vi "SQL.TestData.vi"(3 "最大查询天数":u32, 5 "单项查询索引":i32, 6 "error in (no error)":errorcluster, 7 "Folder Path":path caption="文件夹路径", 8 "Result":string, 9 "Serial_number":string, 10 "Time":string, 11 "Date":string) -> (0 "SQL Results":string[][](table)=[["1.Audio RX", "91.081303", "2.Audio TX", "0.095270", "20121122", "13:32:50", "1170000000689", "PASS"], ["1.Audio RX", "91.143105", "2.Audio TX", "0.095494", "20121122", "13:39:33", "1170000000689", "PASS"], ["1.Audio RX", "91.991153", "2.Audio TX", "0.100831", "20121122", "13:54:04", "1111111111111", "PASS"], ["1.Audio RX", "91.857442", "2.Audio TX", "0.105589", "20121122", "13:56:23", "1172000000041", "PASS"], ["1.Audio RX", "92.085102", "2.Audio TX", "0.101190", "20121122", "13:57:37", "1172000000027", "PASS"], ["1.Audio RX", "91.878361", "2.Audio TX", "0.100191", "20121122", "13:59:11", "1172000000362", "PASS"], ["1.Audio RX", "92.029742", "2.Audio TX", "0.098333", "20121122", "14:02:06", "1172000000287", "PASS"], ["1.Audio RX", "91.480339", "2.Audio TX", "0.101565", "20121122", "14:04:55", "1170000000436", "PASS"], ["1.Audio RX", "91.969090", "2.Audio TX", "0.101169", "20121122", "14:06:27", "1172000000171", "PASS"], ["1.Audio RX", "92.221462", "2.Audio TX", "0.099581", "20121122", "14:09:34", "1172000000034", "PASS"], ["1.Audio RX", "91.987652", "2.Audio TX", "0.098084", "20121122", "14:11:36", "1172000000317", "PASS"], ["1.Audio RX", "92.074553", "2.Audio TX", "0.099366", "20121122", "14:13:21", "1172000000263", "PASS"], ["1.Audio RX", "92.132843", "2.Audio TX", "0.098619", "20121122", "14:14:51", "1172000000492", "PASS"], ["1.Audio RX", "92.082562", "2.Audio TX", "0.099291", "20121122", "14:16:15", "1172000000010", "PASS"], ["1.Audio RX", "91.950055", "2.Audio TX", "0.100073", "20121122", "14:17:31", "1172000000041", "PASS"], ["1.Audio RX", "92.103586", "2.Audio TX", "0.100658", "20121122", "14:28:07", "0000000000000", "PASS"], ["1.Audio RX", "92.130135", "2.Audio TX", "0.099393", "20121122", "14:31:21", "1172000000331", "PASS"], ["1.Audio RX", "92.260601", "2.Audio TX", "0.099085", "20121122", "14:33:09", "1172000000416", "PASS"], ["1.Audio RX", "91.917260", "2.Audio TX", "0.099118", "20121122", "14:34:45", "1172000000294", "PASS"], ["1.Audio RX", "91.905751", "2.Audio TX", "0.097974", "20121122", "14:36:10", "1172000000423", "PASS"], ["1.Audio RX", "92.133605", "2.Audio TX", "0.097918", "20121122", "14:37:41", "1172000000119", "PASS"], ["1.Audio RX", "92.096734", "2.Audio TX", "0.102493", "20121122", "14:40:09", "1172000000508", "PASS"], ["1.Audio RX", "92.042766", "2.Audio TX", "0.097988", "20121122", "14:41:47", "1172000000157", "PASS"], ["1.Audio RX", "92.072530", "2.Audio TX", "0.098405", "20121122", "14:42:41", "1172000000157", "PASS"], ["1.Audio RX", "91.988608", "2.Audio TX", "0.100953", "20121122", "14:45:30", "1172000000164", "PASS"], ["1.Audio RX", "92.115288", "2.Audio TX", "0.099866", "20121122", "14:46:43", "1172000000379", "PASS"], ["1.Audio RX", "91.931552", "2.Audio TX", "0.098401", "20121122", "14:48:07", "1172000000201", "PASS"], ["1.Audio RX", "92.141466", "2.Audio TX", "0.102419", "20121122", "14:49:20", "1172000000324", "PASS"], ["1.Audio RX", "91.932576", "2.Audio TX", "0.099878", "20121122", "14:51:57", "1172000000355", "PASS"], ["1.Audio RX", "92.147045", "2.Audio TX", "0.096185", "20121122", "14:54:23", "1172000000133", "PASS"], ["1.Audio RX", "92.010262", "2.Audio TX", "0.097653", "20121122", "14:55:55", "1172000000270", "PASS"], ["1.Audio RX", "92.200920", "2.Audio TX", "0.099317", "20121122", "14:57:32", "1172000000065", "PASS"], ["1.Audio RX", "92.066286", "2.Audio RX", "91.980270", "20121122", "15:11:29", "", "PASS"], ["1.Audio RX", "92.152783", "2.Audio RX", "92.048697", "20121122", "15:14:00", "", "PASS"], ["1.Audio RX", "92.058673", "2.Audio TX", "0.099819", "20121122", "15:54:48", "1170000000689", "PASS"], ["1.Audio RX", "91.953046", "2.Audio TX", "0.099171", "20121122", "15:58:55", "1170000000436", "PASS"]], 1 "单项数据结果":string[](array[string]), 4 "error out":errorcluster)   [LabVIEW 2012, in "Lib_UEL.ATE.lvlib" / "Lib_SQL.lvlib"]
uses:
  Lib_SQL.lvlib
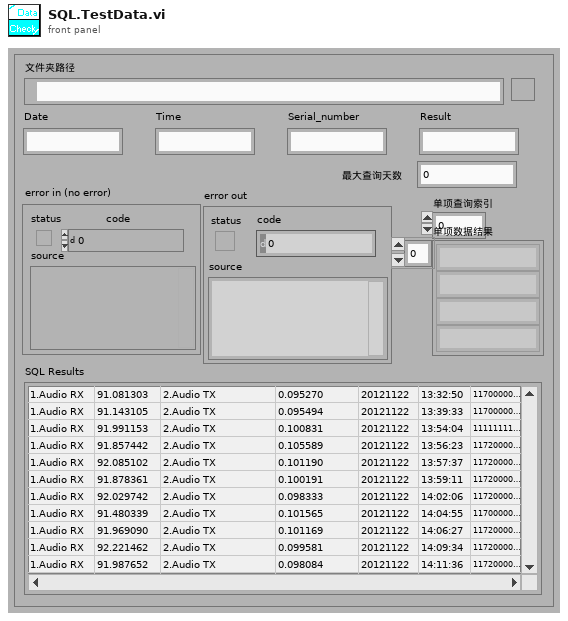
[diagram p1: front panel]
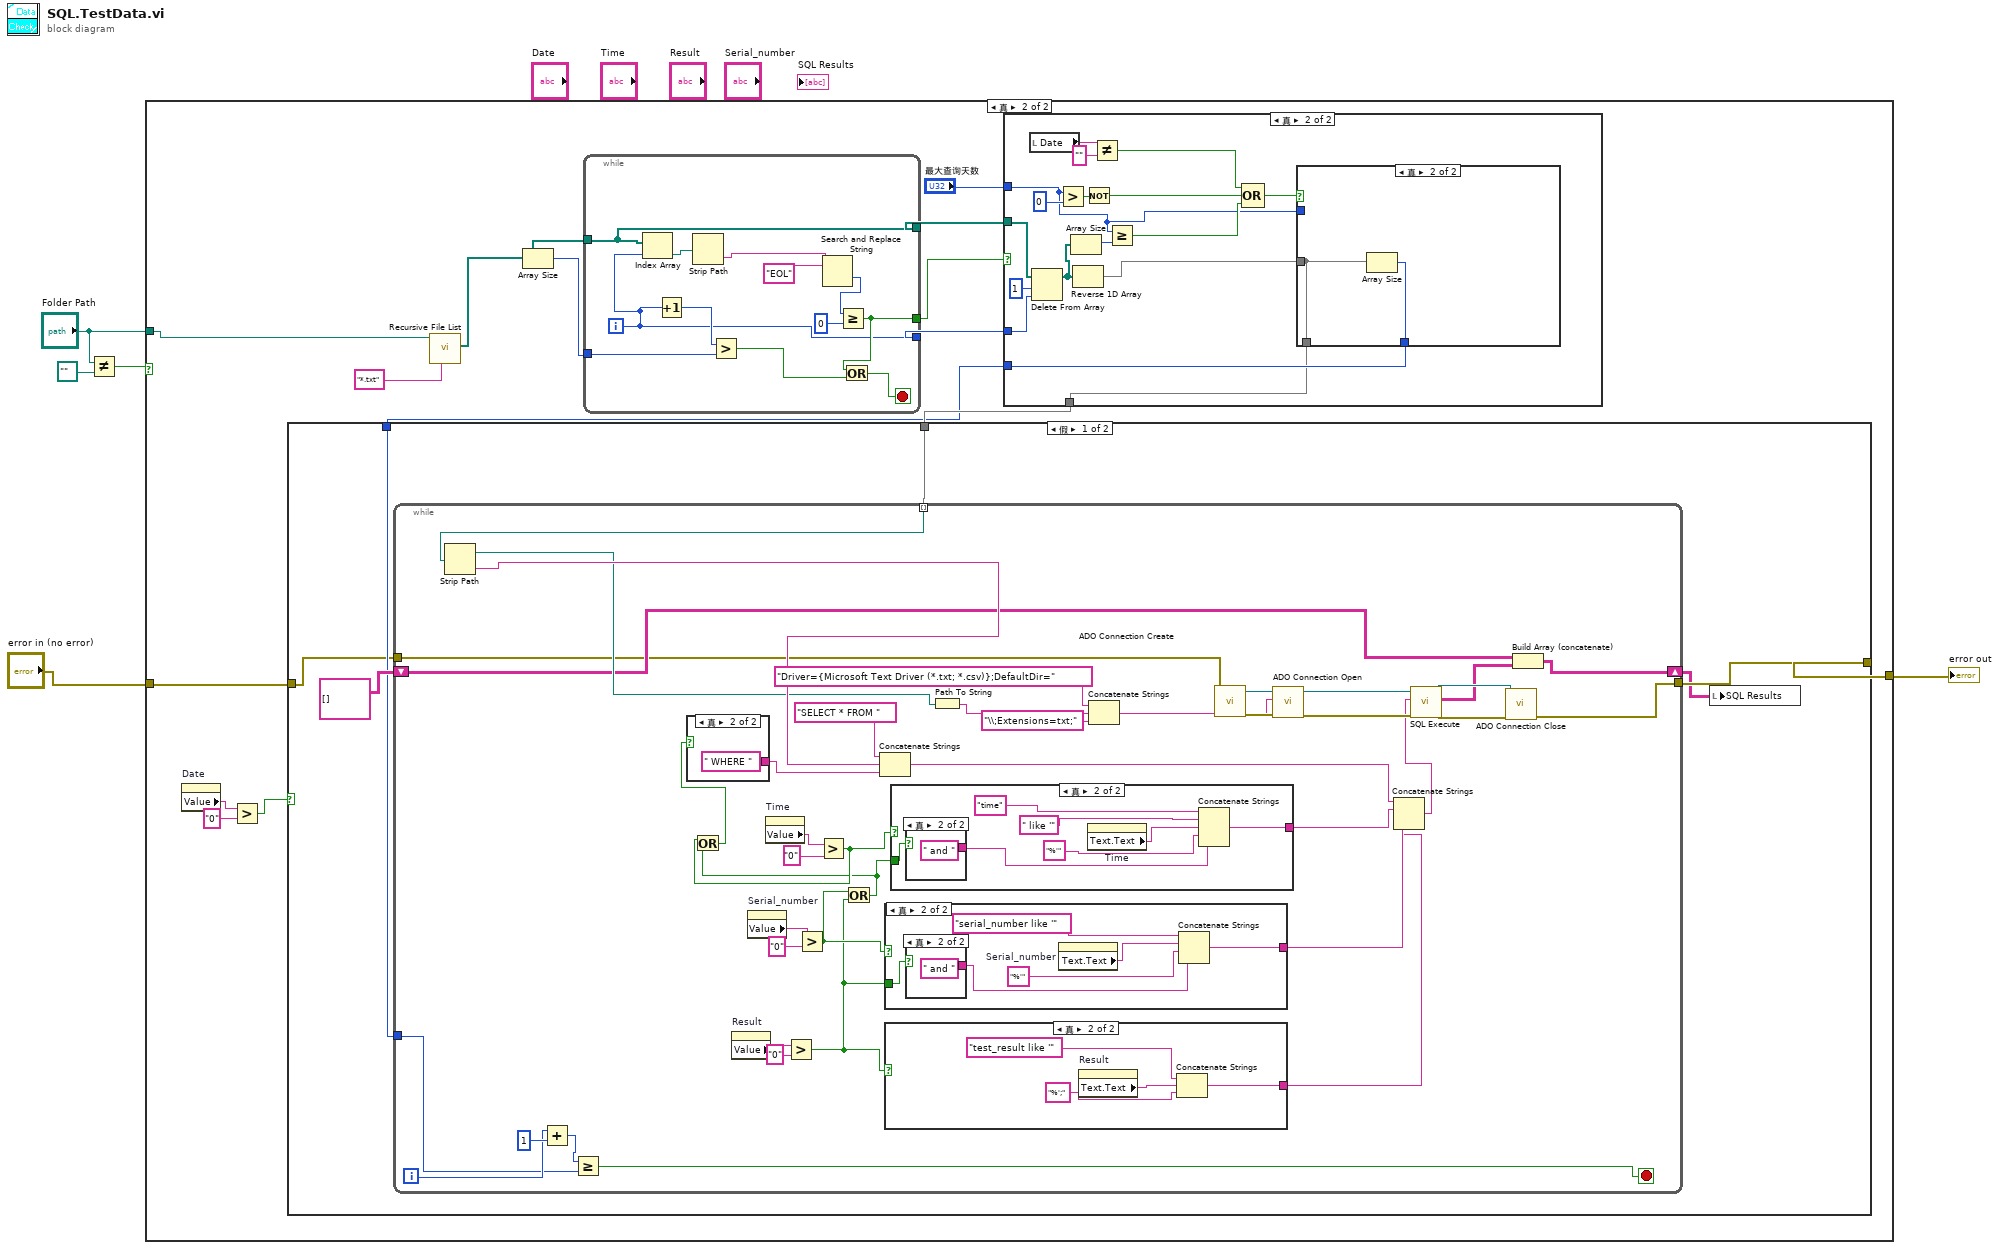
[diagram p0: block diagram]
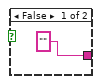
[diagram p3: hidden frame]
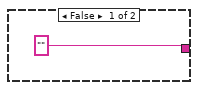
[diagram p4: hidden frame]
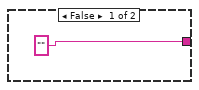
[diagram p5: hidden frame]
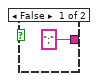
[diagram p6: hidden frame]
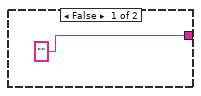
[diagram p7: hidden frame]
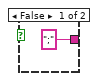
[diagram p8: hidden frame]
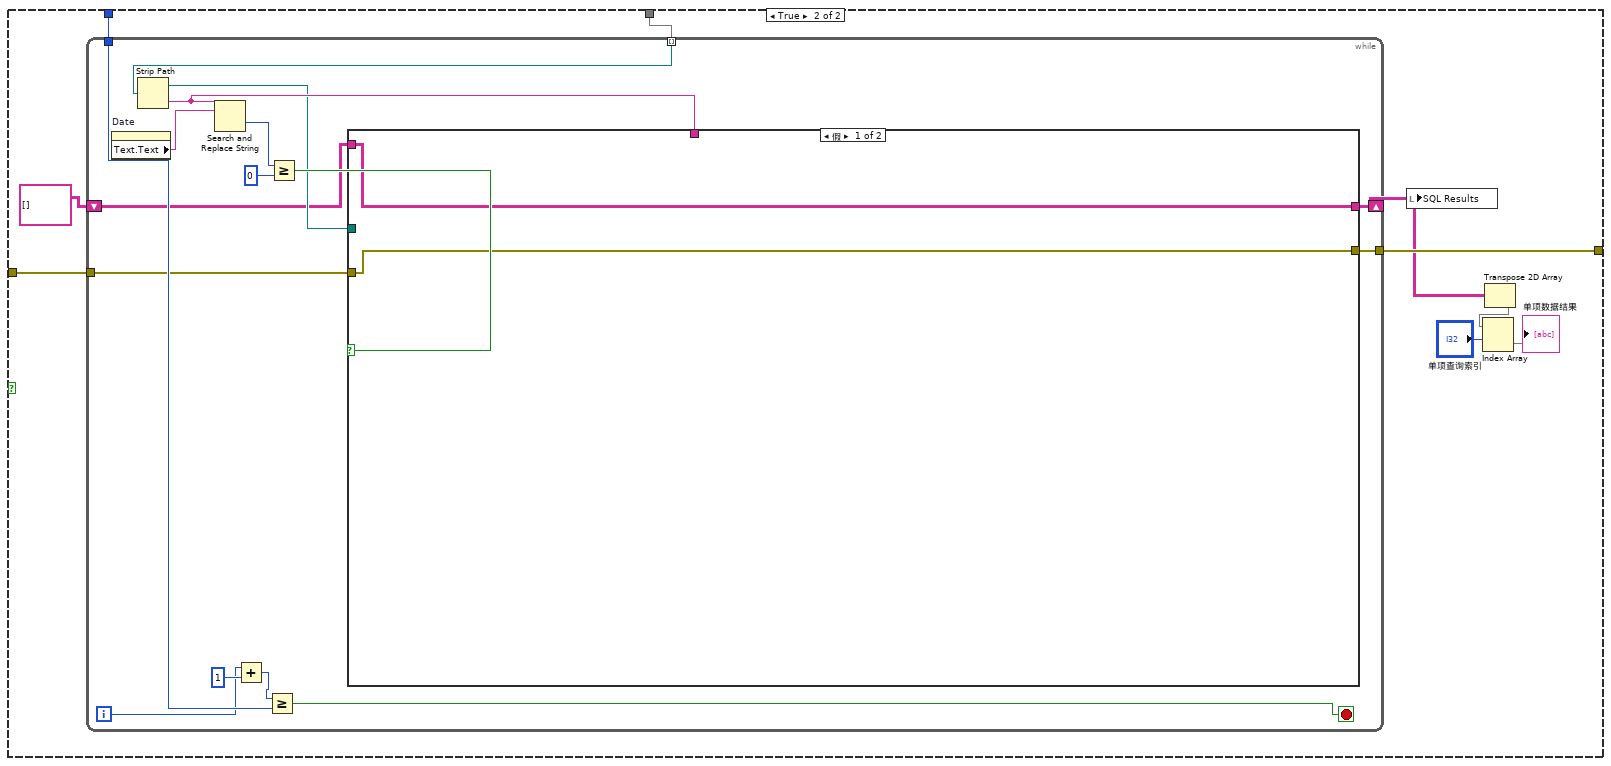
[diagram p9: hidden frame]
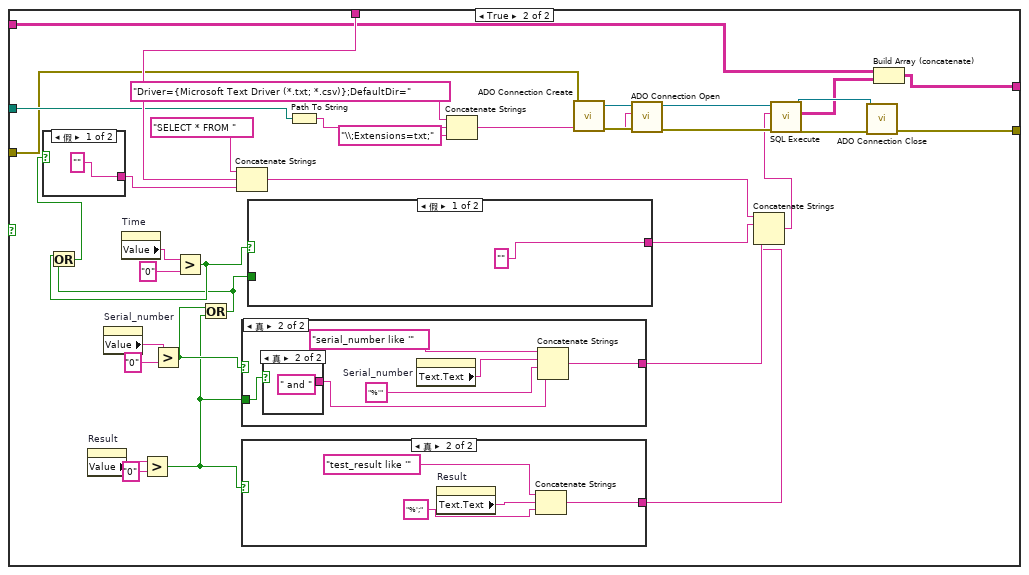
[diagram p10: hidden frame]
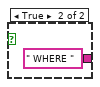
[diagram p11: hidden frame]
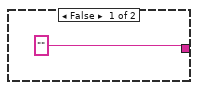
[diagram p12: hidden frame]
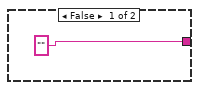
[diagram p13: hidden frame]
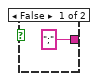
[diagram p14: hidden frame]
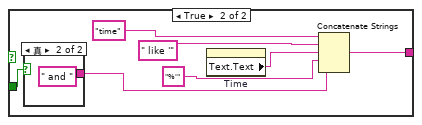
[diagram p15: hidden frame]
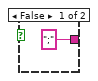
[diagram p16: hidden frame]
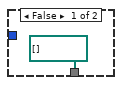
[diagram p17: hidden frame]
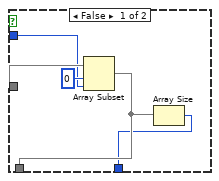
[diagram p18: hidden frame]
diagram:
  n1 = Not Equal?(x="Folder Path", y=path "") -> (x != y?=w1:bool)
  n2 = case shown="真" w1 {
    tunnel: "Folder Path" -> [_ w21]
    tunnel: [w6 w11] -> w5
    tunnel: "error in (no error)" -> [w6 w9]
    frame False {
    }
    frame True {
      n3 = property on="Date" class="Str"() -> ("Value"=w15:string)  [unwired: 2 in, 2 out]
      n4 = Greater?(x=w15, y="0") -> (0:w13:bool)
      n5 = call <vilib>:"Recursive File List.vi"("pattern"="*.txt", "Folder Path"=w21) -> ("All Files in Dir"=w8:path[])  [unwired: 5 in, 4 out]
      n6 = Array Size(array=w8) -> (size(s)=w7:i32)
      n7 = while {
        tunnel: w8 -> [w211]
        tunnel: [w211] -> w19
        tunnel: w7 -> [w210]
        tunnel: [w209] -> w18
        tunnel: [w208] -> w17
        i -> [w208]
        stop <- w212 stop-if-true
        n8 = Index Array(array=w211, index=w208) -> (element=w214:path)
        n9 = Increment(x=w208) -> (x+1=w218:i32)
        n10 = Strip Path(path=w214) -> (name=w213:string)  [unwired: 1 out]
        n11 = Greater?(x=w218, y=w210) -> (0:w215:bool)
        n12 = Search and Replace String(input string=w213, search string="EOL" ("搜索字符串")) -> (offset past replacement=w217:i32)  [unwired: 6 in, 3 out]
        n13 = Greater Or Equal?(x=w217, y=0) -> (x >= y?=w209:bool)
        n14 = Or(x=w209, y=w215) -> (x .or. y?=w212:bool)
      }
      n15 = case shown="真" w18 {
        tunnel: w19 -> [_ w199]
        tunnel: w17 -> [_ w198]
        tunnel: [path[] [] ("All Files in Dir") w195] -> w16
        tunnel: [_ w197] -> w12
        tunnel: "最大查询天数" -> [_ w187]
        frame False {
        }
        frame True {
          n16 = local read "Date"() -> (w186:string)
          n17 = Delete From Array(array=w199, length=1 ("长度"), index=w198) -> (array with subset deleted=w193:path[])  [unwired: 1 out]
          n18 = Greater?(x=w187, y=u32 0) -> (0:w189:bool)
          n19 = Array Size(array=w193) -> (size(s)=w192:i32)
          n20 = Reverse 1D Array(array=w193) -> (reversed array=w194:path[])
          n21 = Not(x=w189) -> (.not. x?=w188:bool)
          n22 = Not Equal?(x=w186, y="") -> (x != y?=w184:bool)
          n23 = Greater Or Equal?(x=w187, y=w192) -> (x >= y?=w190:bool)
          n24 = Compound Arithmetic op=OR(w184, w188, w190) -> (w191:bool)
          n25 = case shown="真" w191 {
            tunnel: w194 -> [w205 w206]
            tunnel: [w201 w207] -> w197
            tunnel: [w202 w206] -> w195
            tunnel: w187 -> [w203 _]
            frame False {
              n26 = Array Subset(array=w205, index=0 ("索引"), length=w203) -> (w202:path[])
              n27 = Array Size(array=w202) -> (size(s)=w201:i32)
            }
            frame True {
              n28 = Array Size(array=w206) -> (size(s)=w207:i32)
            }
          }
        }
      }
      n29 = case shown="假" w13 {
        tunnel: w16 -> [w26 w103]
        tunnel: w12 -> [w25 w102]
        tunnel: [w24 w100] -> w11
        tunnel: w9 -> [w23 w99]
        frame False {
          n30 = while {
            tunnel: w26 -> [w67] mode=indexing
            shift-right: [w60] -> w22
            shift-left: string[][] [] ("Data") -> [w61]
            tunnel: w25 -> [w59]
            tunnel: [w29] -> w24
            tunnel: w23 -> [w28]
            i -> [w63]
            stop <- w64 stop-if-true
            n31 = Strip Path(path=w67) -> (stripped path=w62:path, name=w68:string)
            n32 = Add(x=w63, y=1) -> (x+y=w66:i32)
            n33 = Greater Or Equal?(x=w66, y=w59) -> (x >= y?=w64:bool)
            n34 = property on="Result" class="Str"() -> ("Value"=w43:string)  [unwired: 2 in, 2 out]
            n35 = property on="Serial_number" class="Str"() -> ("Value"=w45:string)  [unwired: 2 in, 2 out]
            n36 = property on="Time" class="Str"() -> ("Value"=w47:string)  [unwired: 2 in, 2 out]
            n37 = Greater?(x=w43, y="0") -> (0:w34:bool)
            n38 = Greater?(x=w45, y="0") -> (0:w35:bool)
            n39 = Greater?(x=w47, y="0") -> (0:w32:bool)
            n40 = Or(x=w35, y=w34) -> (x .or. y?=w31:bool)
            n41 = Or(x=w32, y=w31) -> (x .or. y?=w33:bool)
            n42 = case shown="真" w33 {
              tunnel: ["" " WHERE "] -> w41
              frame False {
              }
              frame True {
              }
            }
            n43 = Concatenate Strings("SELECT * FROM ", w68, w41) -> (w40:string)
            n44 = case shown="真" w35 {
              tunnel: ["" w78] -> w38
              tunnel: w34 -> [_ w77]
              frame False {
              }
              frame True {
                n45 = case shown="真" w77 {
                  tunnel: [";" " and "] -> w79
                  frame False {
                  }
                  frame True {
                  }
                }
                n46 = property on="Serial_number" class="Str"() -> ("Text.Text"=w81:string)  [unwired: 2 in, 2 out]
                n47 = Concatenate Strings("serial_number like '", w81, "%'", w79) -> (w78:string)
              }
            }
            n48 = case shown="真" w34 {
              tunnel: ["" w72] -> w37
              frame False {
              }
              frame True {
                n49 = property on="Result" class="Str"() -> ("Text.Text"=w74:string)  [unwired: 2 in, 2 out]
                n50 = Concatenate Strings("test_result like '", w74, "%';") -> (w72:string)
              }
            }
            n51 = case shown="真" w32 {
              tunnel: ["" w87] -> w39
              tunnel: w31 -> [_ w86]
              frame False {
              }
              frame True {
                n52 = case shown="真" w86 {
                  tunnel: [";" " and "] -> w88
                  frame False {
                  }
                  frame True {
                  }
                }
                n53 = property on="Time" class="Str"() -> ("Text.Text"=w90:string)  [unwired: 2 in, 2 out]
                n54 = Concatenate Strings("time", " like '", w90, "%'", w88) -> (w87:string)
              }
            }
            n55 = Path To String(path=w62) -> (string=w50:string)
            n56 = Concatenate Strings("Driver={Microsoft Text Driver (*.txt; *.csv)};DefaultDir=", w50, "\\;Extensions=txt;" ("字符串")) -> (w48:string)
            n57 = call <userlib>:"ADO Connection Create.vi"("error in (no error)"=w28) -> ("error out"=w56:errorcluster, "ADODB._Connection Out"=w57:refnum<k7>)  [unwired: 9 in]
            n58 = call <userlib>:"ADO Connection Open.vi"("error in (no error)"=w56, "ConnectionString"=w48, "ADODB._Connection In"=w57) -> ("error out"=w54:errorcluster, "ADODB._Connection Out"=w55:refnum<k7>)  [unwired: 7 in]
            n59 = Concatenate Strings(w40, w39, w38, w37) -> (w36:string)
            n60 = call <userlib>:"SQL Execute.vi"("error in (no error)"=w54, "Command Text"=w36, "ADODB._Connection In"=w55) -> ("error out"=w53:errorcluster, "Data"=w30:string[][], "ADODB._Connection Out"=w52:refnum<k7>)  [unwired: 5 in, 1 out]
            n61 = call <userlib>:"ADO Connection Close.vi"("error in (no error)"=w53, "ADODB._Connection In"=w52) -> ("error out"=w29:errorcluster)  [unwired: 8 in, 1 out]
            n62 = Build Array (concatenate)(w61, w30) -> (w60:string[][])
          }
          n63 = local write "SQL Results"(w22) -> ()
        }
        frame True {
          n64 = while {
            tunnel: w103 -> [w116] mode=indexing
            tunnel: w102 -> [w115]
            shift-right: [w106] -> w95
            shift-left: string[][] [] ("Data") -> [w107]
            tunnel: [w105] -> w100
            tunnel: w99 -> [w104]
            i -> [w109]
            stop <- w110 stop-if-true
            n65 = property on="Date" class="Str"() -> ("Text.Text"=w114:string)  [unwired: 2 in, 2 out]
            n66 = Strip Path(path=w116) -> (stripped path=w108:path, name=w117:string)
            n67 = Search and Replace String(input string=w117, search string=w114) -> (offset past replacement=w119:i32)  [unwired: 6 in, 3 out]
            n68 = Add(x=w109, y=1) -> (x+y=w112:i32)
            n69 = Greater Or Equal?(x=w112, y=w115) -> (x >= y?=w110:bool)
            n70 = Greater Or Equal?(x=w119, y=0) -> (x >= y?=w118:bool)
            n71 = case shown="假" w118 {
              tunnel: w117 -> [_ w155]
              tunnel: w108 -> [_ w127]
              tunnel: [w121 w124] -> w106
              tunnel: w107 -> [w121 w126]
              tunnel: [w120 w123] -> w105
              tunnel: w104 -> [w120 w122]
              frame False {
              }
              frame True {
                n72 = property on="Result" class="Str"() -> ("Value"=w140:string)  [unwired: 2 in, 2 out]
                n73 = property on="Serial_number" class="Str"() -> ("Value"=w142:string)  [unwired: 2 in, 2 out]
                n74 = property on="Time" class="Str"() -> ("Value"=w144:string)  [unwired: 2 in, 2 out]
                n75 = Greater?(x=w140, y="0") -> (0:w131:bool)
                n76 = Greater?(x=w142, y="0") -> (0:w132:bool)
                n77 = Greater?(x=w144, y="0") -> (0:w129:bool)
                n78 = Or(x=w132, y=w131) -> (x .or. y?=w128:bool)
                n79 = Or(x=w129, y=w128) -> (x .or. y?=w130:bool)
                n80 = case shown="假" w130 {
                  tunnel: ["" " WHERE "] -> w138
                  frame False {
                  }
                  frame True {
                  }
                }
                n81 = Concatenate Strings("SELECT * FROM ", w155, w138) -> (w137:string)
                n82 = case shown="真" w132 {
                  tunnel: ["" w166] -> w135
                  tunnel: w131 -> [_ w165]
                  frame False {
                  }
                  frame True {
                    n83 = case shown="真" w165 {
                      tunnel: [";" " and "] -> w167
                      frame False {
                      }
                      frame True {
                      }
                    }
                    n84 = property on="Serial_number" class="Str"() -> ("Text.Text"=w169:string)  [unwired: 2 in, 2 out]
                    n85 = Concatenate Strings("serial_number like '", w169, "%'", w167) -> (w166:string)
                  }
                }
                n86 = case shown="真" w131 {
                  tunnel: ["" w160] -> w134
                  frame False {
                  }
                  frame True {
                    n87 = property on="Result" class="Str"() -> ("Text.Text"=w162:string)  [unwired: 2 in, 2 out]
                    n88 = Concatenate Strings("test_result like '", w162, "%';") -> (w160:string)
                  }
                }
                n89 = case shown="假" w129 {
                  tunnel: ["" w175] -> w136
                  tunnel: w128 -> [_ w174]
                  frame False {
                  }
                  frame True {
                    n90 = case shown="真" w174 {
                      tunnel: [";" " and "] -> w176
                      frame False {
                      }
                      frame True {
                      }
                    }
                    n91 = property on="Time" class="Str"() -> ("Text.Text"=w178:string)  [unwired: 2 in, 2 out]
                    n92 = Concatenate Strings("time", " like '", w178, "%'", w176) -> (w175:string)
                  }
                }
                n93 = Path To String(path=w127) -> (string=w147:string)
                n94 = Concatenate Strings("Driver={Microsoft Text Driver (*.txt; *.csv)};DefaultDir=", w147, "\\;Extensions=txt;" ("字符串")) -> (w145:string)
                n95 = call <userlib>:"ADO Connection Create.vi"("error in (no error)"=w122) -> ("error out"=w153:errorcluster, "ADODB._Connection Out"=w154:refnum<k7>)  [unwired: 9 in]
                n96 = call <userlib>:"ADO Connection Open.vi"("error in (no error)"=w153, "ConnectionString"=w145, "ADODB._Connection In"=w154) -> ("error out"=w151:errorcluster, "ADODB._Connection Out"=w152:refnum<k7>)  [unwired: 7 in]
                n97 = Concatenate Strings(w137, w136, w135, w134) -> (w133:string)
                n98 = call <userlib>:"SQL Execute.vi"("error in (no error)"=w151, "Command Text"=w133, "ADODB._Connection In"=w152) -> ("error out"=w150:errorcluster, "Data"=w125:string[][], "ADODB._Connection Out"=w149:refnum<k7>)  [unwired: 5 in, 1 out]
                n99 = call <userlib>:"ADO Connection Close.vi"("error in (no error)"=w150, "ADODB._Connection In"=w149) -> ("error out"=w123:errorcluster)  [unwired: 8 in, 1 out]
                n100 = Build Array (concatenate)(w126, w125) -> (w124:string[][])
              }
            }
          }
          n101 = local write "SQL Results"(w95) -> ()
          n102 = Transpose 2D Array(2D array=w95) -> (transposed array=w96:string[][])
          n103 = Index Array(array=w96, index (row)="单项查询索引") -> (element=→"单项数据结果":string[])  [unwired: 1 in]
        }
      }
    }
  }
  "error out" <- w5
